vi "Identify.vi"(8 "error in (no error)":errorcluster, 11 "Abort Keep Alive in":refnum<class "Abort Keep Alive.lvclass">) -> (0 "error out":errorcluster, 2 "Plugin is Valid":bool, 3 "Abort Keep Alive out":refnum<class "Abort Keep Alive.lvclass">)   [LabVIEW 2018, in "Abort Keep Alive.lvlib" / "Abort Keep Alive.lvclass"]
uses:
  Abort Keep Alive.lvclass
  C:/Sequence Automation/Plugins/Measurement Interface.lvlibp/Measurement Interface.lvclass
  Plugins/Measurement Interface.lvlibp/Private Methods/Measurement Definition Entry/Read Measurement Definition Entry.vi
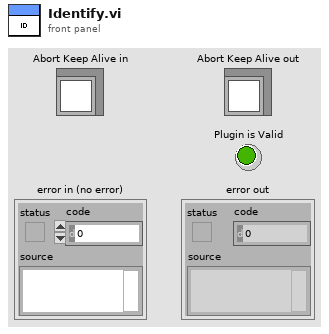
[diagram p1: front panel]
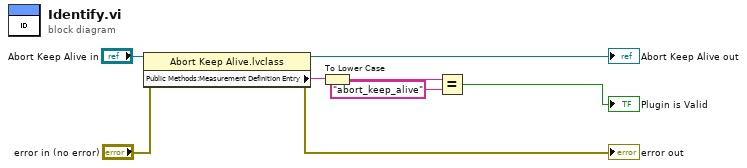
[diagram p0: block diagram]
diagram:
  n1 = property class="Abort Keep Alive.lvclass"(reference="Abort Keep Alive in", error in="error in (no error)") -> (reference out=→"Abort Keep Alive out":refnum<class "Abort Keep Alive.lvclass">, error out=→"error out":errorcluster, "Public Methods:Measurement Definition Entry"=w4:string)
  n2 = To Lower Case(string=w4) -> (all lower case string=w3:string)
  n3 = Equal?(x=w3, y="abort_keep_alive") -> (x = y?=→"Plugin is Valid":bool)
